vi "SimpleMotorFF_MaxAchieveAccel.vi"(9 "Velocity":dbl, 10 "MaxVoltage":dbl, 11 "SIMPLE_MOTOR_FF":T1 {"KnInv" format="%13.4f"; "Ka" format="%13.4f"; "Kv" format="%13.4f"; "Ks" format="%13.4f"}) -> (3 "MaxAccel":dbl)   [LabVIEW 2019, in "Trajectory_Library.lvlib"]
doc: "Calculates the maximum achievable acceleration given a maximum voltage supply and a velocity. Useful for ensuring that velocity and acceleration constraints for a trapezoidal profile are simultaneously achievable - enter the velocity constraint, and this will give you a simultaneously-achievable acceleration constraint.\n\nParameters:\n - Simple_Motor_FF - Data structure containing constants\n - maxVoltage -The maximum voltage that can be supplied to the motor.\n - velocity - The velocity of the motor.\n\nReturns:\n MaxAccel - The maximum possible acceleration at the given velocity."
uses:
  Trajectory_Library.lvlib
  TypeDef/SIMPLE_MOTOR_FF.ctl
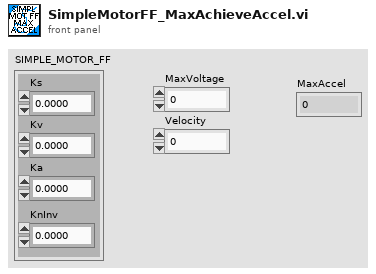
[diagram p1: front panel]
types:
  T1 = typedef "Trajectory_Library.lvlib/SIMPLE_MOTOR_FF.ctl" = cluster{"Ks":dbl, "Kv":dbl, "Ka":dbl, "KnInv":dbl}
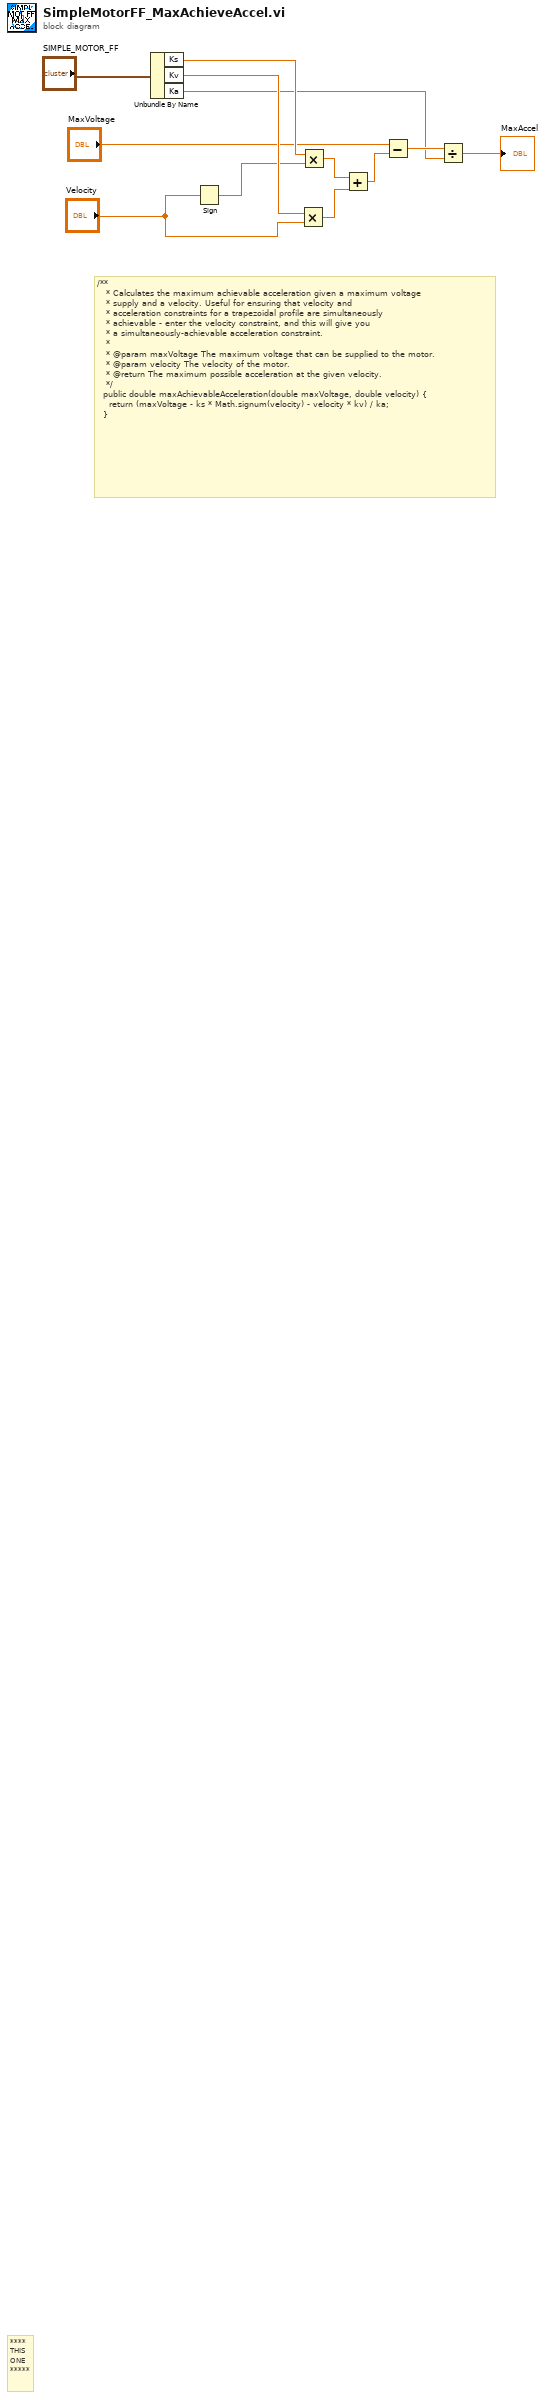
[diagram p0: block diagram]
diagram:
  # "/**\n   * Calculates the maximum achievable acceleration given a maximum voltage\n   * supply and a velocity. Useful for ensuring that velocity and\n   * acceleration constraints for a trapezoidal profile are simultaneously\n   * achievable - enter the velocity constraint, and this will give you\n   * a simultaneously-achievable acceleration constraint.\n   *\n   * @param maxVoltage The maximum voltage that can be supplied to the motor.\n   * @param velocity The velocity of the motor.\n   * @return The maximum possible acceleration at the given velocity.\n   */\n  public double maxAchievableAcceleration(double maxVoltage, double velocity) {\n    return (maxVoltage - ks * Math.signum(velocity) - velocity * kv) / ka;\n  }"
  # "****\nTHIS\nONE\n*****"
  n1 = Unbundle By Name("SIMPLE_MOTOR_FF") -> ("Ks"=w11:dbl, "Kv"=w10:dbl, "Ka"=w2:dbl)
  n2 = Sign(1:"Velocity") -> (0:w8:dbl)
  n3 = Multiply(x=w10, y="Velocity") -> (x*y=w5:dbl)
  n4 = Multiply(x=w11, y=w8) -> (x*y=w6:dbl)
  n5 = Add(x=w6, y=w5) -> (x+y=w4:dbl)
  n6 = Subtract(x="MaxVoltage", y=w4) -> (x-y=w3:dbl)
  n7 = Divide(x=w3, y=w2) -> (x/y=→"MaxAccel":dbl)
